vi "Set configuration chain.vi"(8 "error in (no error)":errorcluster, 9 "class names":string[](array[string]), 10 "configuration":variant[](array[variant]), 11 "ExampleClassC in":refnum<class "ExampleClassC.lvclass">) -> (0 "error out":errorcluster, 3 "ExampleClassC out":refnum<class "ExampleClassC.lvclass">)   [LabVIEW 2012, in "ExampleClassC.lvclass"]
uses:
  ExampleClassC.lvclass
  <vilib>/Distrio/Murmex/Murmex/Murmex.lvclass
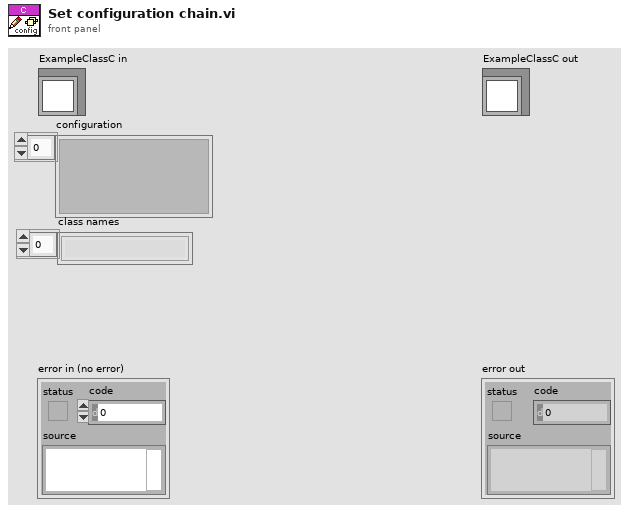
[diagram p1: front panel]
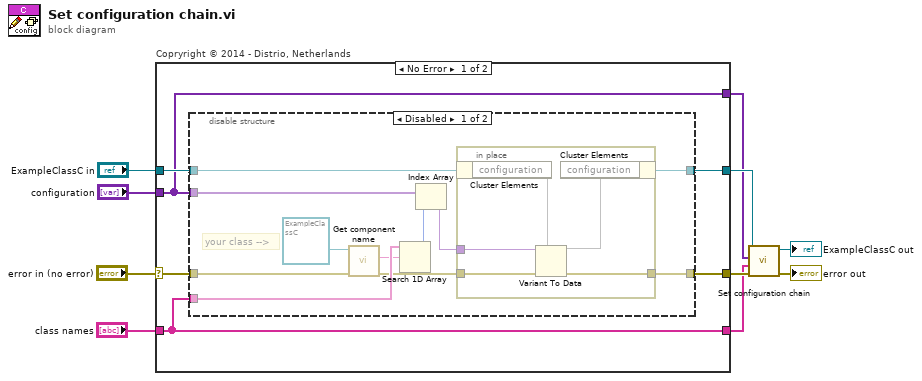
[diagram p0: block diagram]
diagram:
  n1 = case "Copryright © 2014 - Distrio, Netherlands" shown="No Error" "error in (no error)" {
    selector: "error in (no error)" -> [w16 w36]
    tunnel: [w13 w36] -> w5
    tunnel: [w14 w35] -> w4
    tunnel: "ExampleClassC in" -> [w15 w35]
    tunnel: "class names" -> [w11 _]
    tunnel: "configuration" -> [w12 _]
    tunnel: [w12 _] -> w2
    tunnel: [w11 _] -> w1
    frame No Error {
      n2 = disable-structure shown="Disabled" {
        disable-tunnel: w16 -> [w27 w33]
        disable-tunnel: w11 -> [w26 _]
        disable-tunnel: w12 -> [w24 _]
        disable-tunnel: w15 -> [w18 w34]
        disable-tunnel: [w20 w34] -> w14
        disable-tunnel: [w19 w33] -> w13
        frame Disabled {
          # "your class -->"
          n3 = call <vilib>:"Get component name.vi"("error in (no error)"=w27, "Murmex in"=refnum<class "ExampleClassC.lvclass"> refnum ("ExampleClassC in")) -> ("error out"=w21:errorcluster, "component name"=w25:string)  [unwired: 7 in, 1 out]
          n4 = Search 1D Array(1D array=w26, element=w25) -> (index of element=w23:i32)  [unwired: 1 in]
          n5 = Index Array(array=w24, index=w23) -> (element=w22:variant)
          n6 = in-place {
            in-place-border: w22 -> [w32]
            in-place-border: w21 -> [w30]
            in-place-border: [w28] -> w19
            n7 = in-place-cluster #1(w18) -> ("configuration"=w31)
            n8 = Variant To Data(error in=w30, type=w31, Variant=w32) -> (data=w29, error out=w28:errorcluster)
            n9 = in-place-cluster #1("configuration"=w29) -> (w20:refnum<class "ExampleClassC.lvclass">)
          }
        }
        frame Enabled {
        }
      }
    }
    frame Error {
    }
  }
  n10 = call-parent "Set configuration chain.vi"("error in (no error)"=w5, "class names"=w1, "configuration"=w2, "Murmex in"=w4) -> ("error out"=→"error out":errorcluster, "Murmex out"=→"ExampleClassC out":refnum<class "ExampleClassC.lvclass">)  [unwired: 6 in]
